vi "GetOneErrorData.vi"(8 "ErrorIn":errorcluster caption="Error In(no Error)", 9 "ErrorCode":i32, 11 "ReferenceIn":refnum<class "ErrorDefinitionSQLite.lvclass"> caption="Reference In") -> (0 "ErrorOut":errorcluster caption="Error Out", 1 "Library":string, 2 "Text":string, 3 "ReferenceOut":refnum<class "ErrorDefinitionSQLite.lvclass"> caption="Reference Out", 4 "Description":string)   [LabVIEW 2018, in "ErrorDefinitionSQLite.lvclass"]
uses:
  <userlib>/_express/CustomErrorCreator/ErrorDefinitionSQLite/ErrorDefinitionSQLite.lvclass
  <vilib>/drjdpowell/SQLite Library/SQL Connection/Open (path).vi
  <vilib>/drjdpowell/SQLite Library/SQL Connection/Open (string).vi
  <vilib>/AdvancedString/Path To Command Line String.vi
  <vilib>/drjdpowell/SQLite Library/SQL Connection/Execute SQL.vi
  <vilib>/drjdpowell/SQLite Library/SQL Connection/Connection.lvclass
  <vilib>/drjdpowell/SQLite Library/SQLite.lvlib
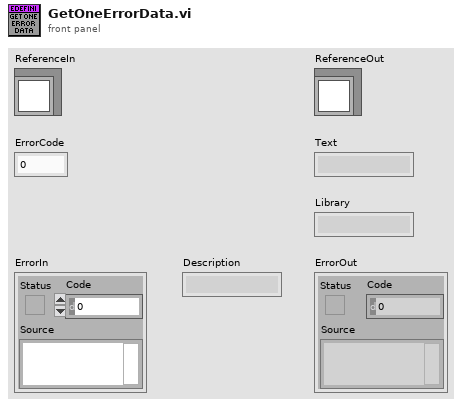
[diagram p1: front panel]
types:
  T1 = enum16{"New or existing", "Existing", "Read only"}
  T2 = typedef "ErrorDefinitionSQLite.lvclass/ObjectAttributes.ctl" = cluster{"Path":path}
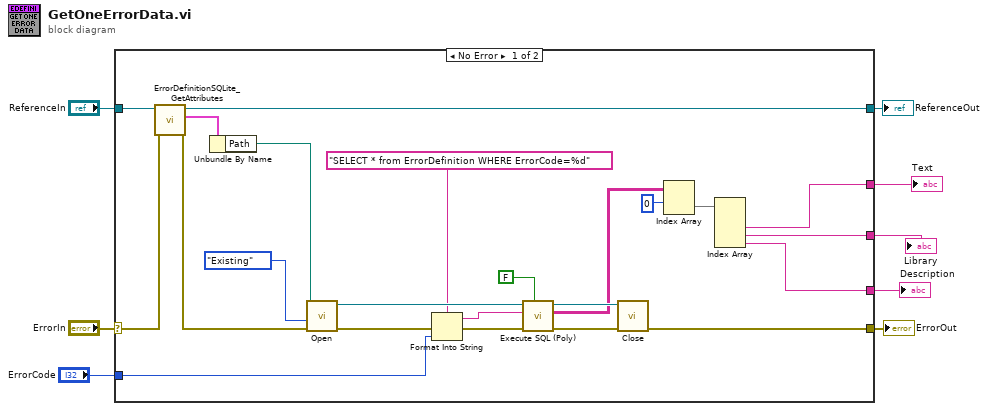
[diagram p0: block diagram]
diagram:
  n1 = case shown="No Error" "ErrorIn" {
    selector: "ErrorIn" -> [w31 w33]
    tunnel: [w15 w33] -> w7
    tunnel: [w29 w32] -> w5
    tunnel: "ReferenceIn" -> [w30 w32]
    tunnel: "ErrorCode" -> [w18 _]
    tunnel: [w11 _] -> w3
    tunnel: [w10 _] -> w2
    tunnel: [w9 _] -> w1
    frame No Error {
      n2 = call <userlib>:"ErrorDefinitionSQLite_GetAttributes.vi"("ErrorIn"=w31, "Reference in"=w30) -> ("ErrorOut"=w25:errorcluster, "Data"=w27:T2, "Reference out"=w29:refnum<class "ErrorDefinitionSQLite.lvclass">)  [unwired: 6 in, 1 out]
      n3 = Unbundle By Name(w27) -> ("Path"=w26:path)
      n4 = call-poly <vilib>:"Open.vi"("error in (no error)"=w25, "File Option"=T1."Existing", "db file"=w26) -> ("error out"=w20:errorcluster, "SQLite Connection"=w23:refnum<class "Connection.lvclass">)  [unwired: 7 in]
      n5 = Format Into String(format string="SELECT * from ErrorDefinition WHERE ErrorCode=%d" ("SQL"), error in=w20, w18) -> (resulting string=w21:string, error out=w19:errorcluster)  [unwired: 1 in]
      n6 = call-poly <vilib>:"Execute SQL (Poly).vi"("Use SAVEPOINT"=FALSE, "error in (no error)"=w19, "SQL"=w21, "SQLite Connection in"=w23) -> ("error out"=w16:errorcluster, "Result Set"=w14:string[][], "SQLite Connection"=w17:refnum<class "Connection.lvclass">)  [unwired: 4 in, 1 out]
      n7 = call-dynamic "Close.vi"("error in (no error)"=w16, "SQLite Connection in"=w17) -> ("error out"=w15:errorcluster)  [unwired: 9 in]
      n8 = Index Array(array=w14, index (row)=0 ("disabled index (col)")) -> (element=w12:string[])  [unwired: 1 in]
      n9 = Index Array(array=w12) -> (element #2=w11:string, element #3=w10:string, element #4=w9:string)  [unwired: 4 in, 1 out]
    }
    frame Error {
    }
  }
  "ErrorOut" <- w7
  "ReferenceOut" <- w5
  "Description" <- w1
  "Library" <- w2
  "Text" <- w3
